vi "Autonomous_Execution.vi"(8 "error in":errorcluster, 9 "Autonomous_Queue":refnum<queue>, 11 "Queue Key":refnum<queue>) -> (2 "Done":bool)   [LabVIEW 2018]
uses:
  Autonomous Utilities/Queue_Key_Data.ctl
  Autonomous Utilities/Robot_Subsystems.ctl
  Subsytems/Drive/Drive_Notifier.ctl
  Subsytems/Drive/Drive_Control_Type.ctl
  Subsytems/Elevator/Elevator_Notifier.ctl
  Subsytems/Elevator/Elevator_Control_Type.ctl
  Subsytems/Elevator/Elevator_Enum_States.ctl
  Subsytems/Climb/Climb_Notifier.ctl
  Subsytems/Climb/Climb_Control_Type.ctl
  Subsytems/Intake_Ball/Intake_Ball_Notifier.ctl
  Subsytems/Intake_Ball/Intake_Ball_Control_Type.ctl
  Subsytems/Intake_Disc/Intake_Disc_Notifier.ctl
  Subsytems/Intake_Disc/Intake_Disc_Control_Type.ctl
  <vilib>/Rock Robotics/WPI/Solenoid/WPI_SolenoidValue.ctl
  Subsytems/Intake_Joint/Intake_Joint_Notifier.ctl
  Subsytems/Intake_Joint/Intake_Joint_Control_Type.ctl
  Subsytems/Intake_Joint/Intake_Joint_Enum_States.ctl
  Global_Variables/Drive_Globals.vi
  Global_Variables/Climb_Globals.vi
  Global_Variables/Elevator_Globals.vi
  Global_Variables/Intake_Joint_Globals.vi
  Global_Variables/Intake_Ball_Globals.vi
  Global_Variables/Intake_Disc_Globals.vi
panel:
  in  "ignore previous (F)":bool
  in  "timeout in ms (-1)":i32=15
  out "notifiers out":refnum<notifier>[](array[refnum])
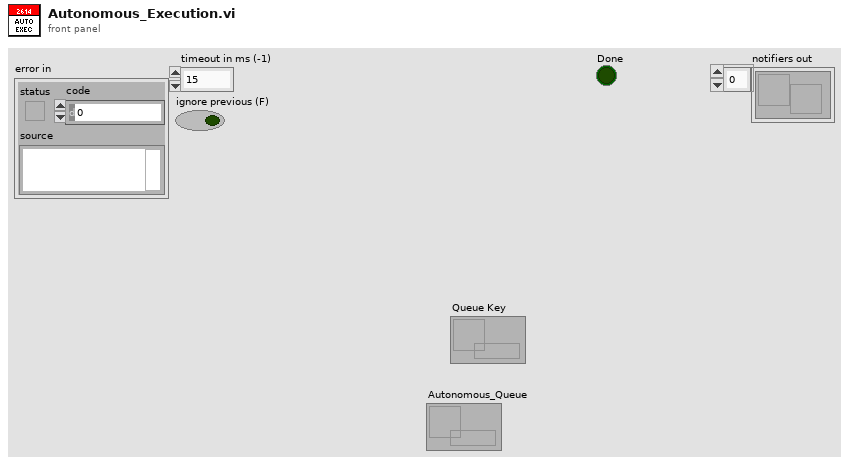
[diagram p1: front panel]
types:
  T1 = typedef "Queue_Key_Data.ctl" = cluster{"Operation Notifier":refnum<notifier>, "Subsystem":string, "Concurrent":bool}
  T2 = typedef "Robot_Subsystems.ctl" = cluster{"Drive Notifier":T3, "Elevator_Notifier":T5, "Climb_Notifier":T8, "Intake_Ball_Notifier":T10, "Intake_Disc_Notifier":T12, "Intake_Joint_Notifier":T15}
  T3 = typedef "Drive_Notifier.ctl" = cluster{"Drive Control List":T4, "Front/Back":dbl, "Left/Right":dbl, "Turn":dbl, "Test_Joy_Y":dbl, "Test_Joy_X":dbl, "Set Wheel Encoder Positions":bool, "Robotcentric":bool, "Reset Gyro":bool, "Rotate Front Right":bool, "Rotate Front Left":bool, "Rotate Back Right":bool, "Rotate Back Left":bool, "Write_Encoder_Positions":bool, "Climb_Advance":bool, "Parameter_One":dbl, "Parameter_Two":dbl, "Parameter_Three":dbl, "Parameter_Four":dbl, "Drive_Notifier":refnum<notifier>, "Step":i32, "Climb_Reverse":bool, "Auto_Target":bool}
  T4 = typedef "Drive_Control_Type.ctl" = enum16{"No_Op", "Write_FL_Position", "Write_FR_Position", "Write_BL_Position", "Write_BR_Position", "Set_Encoder_Positions", "Fieldcentric_PercentVBus", "Fieldcentric", "Robotcentric", "Reset_Gyro", "FR_Wheel", "FL_Wheel", "BR_Wheel", "BL_Wheel", "Drive_Onto_Platform", "Manual_Wheel_Control", "Distance", "Turn_To_Heading", "Turn_To_Target", "Drive_To_Target", "Zero", "Auto_Target", "Drive_Over_Platform", "Heading_Lock", "Time"}
  T5 = typedef "Elevator_Notifier.ctl" = cluster{"Elevator_Control_Type":T6, "Shift":bool, "Brake":bool, "Manual_Lift_Up":bool, "Manual_Lift_Down":bool, "Climb_Advance":bool, "Climb_Reverse":bool, "Low_Rocket":bool, "Mid_Rocket":bool, "High_Rocket":bool, "Cargo_Ship":bool, "Hatch_Floor":bool, "Cargo_Floor":bool, "HP_Hatch":bool, "HP_Cargo":bool, "Depot_Cargo":bool, "Stow":bool, "Set_Position":T7, "Intake_Mode":bool, "Climb_Distance":dbl, "Level_Two":bool, "Parameter_One":dbl, "Parameter_Two":dbl, "Parameter_Three":dbl, "Step":i32, "Elevator_Notifier":refnum<notifier>, "Brake_State":bool, "Shift_State":bool}
  T6 = typedef "Elevator_Control_Type.ctl" = enum16{"No_Op", "Shift", "Brake", "Manual_Elevator_Up", "Manual_Elevator_Down", "Manual_Climb_Up", "Manual_Climb_Down", "Manual_Position_Control", "Elevator_Retract", "Elevator_Extend", "Brake_In_Climb", "Position_Control", "Position", "Shift_Climb"}
  T7 = typedef "Elevator_Enum_States.ctl" = enum16{"Current_Position", "High_Rocket_Hatch_Panel_Floor", "High_Rocket_Hatch_Panel", "Mid_Rocket_Hatch_Panel_Floor", "Mid_Rocket_Hatch_Panel", "Low_Rocket_Hatch_Panel", "Cargo_Ship_Hatch_Panel", "Loading_Station_Hatch_Panel", "Ground_Pickup_Hatch_Panel", "High_Rocket_Cargo", "Mid_Rocket_Cargo", "Low_Rocket_Cargo", "Cargo_Ship_Cargo", "Loading_Station_Cargo", "Ground_Pickup_Cargo", "Depot_Pickup_Cargo", "Descend_Off_Platform", "Stow_Cargo"}
  T8 = typedef "Climb_Notifier.ctl" = cluster{"Climb_Control_Type":T9, "Brake":bool, "Manual_Climb_Up":bool, "Manual_Drive_Forward":bool, "Manual_Drive_Backward":bool, "Manual_Climb_Down":bool, "Climb_Advance":bool, "Climb_Reverse":bool, "Parameter_One":dbl, "Parameter_Two":dbl, "Parameter_Three":dbl, "Step":i32, "Climb_Notifier":refnum<notifier>, "Climb_Distance":dbl, "Level_Two":bool, "Brake_State":bool, "Toggle_Servo":bool}
  T9 = typedef "Climb_Control_Type.ctl" = enum16{"No_Op", "Brake", "Manual_Climb_Up", "Manual_Climb_Down", "Manual_Drive_Forward", "Manual_Drive_Backward", "Back_Wheels_Forward", "Lift_Retract", "Lift_Extend", "Extend_to_Second_Level", "Spin"}
  T10 = typedef "Intake_Ball_Notifier.ctl" = cluster{"Intake_Ball_Control_Type":T11, "Manual_In":bool, "Manual_Out":bool, "Ball_In":bool, "Ball_Out":bool, "Parameter_One":dbl, "Parameter_Two":dbl, "Parameter_Three":dbl, "Step":i32, "Ball_Notifier":refnum<notifier>}
  T11 = typedef "Intake_Ball_Control_Type.ctl" = enum16{"No_Op", "Manual_In", "Manual_Out", "In_Sensor_Stop", "Out_Teleop", "Out", "Stall"}
  T12 = typedef "Intake_Disc_Notifier.ctl" = cluster{"Intake_Disc_Control_Type":T13, "Manual_Disc_Toggle":bool, "Disc_Toggle":bool, "Disc_Toggle_State":bool, "Manual_Press_Toggle":bool, "Disc_Press_State":bool, "Press_Toggle":bool, "Press_Pnuematic":T14, "Disc_Pnuematic":T14, "Disc_Notifier":refnum<notifier>, "Step":i32}
  T13 = typedef "Intake_Disc_Control_Type.ctl" = enum16{"No_Op", "Manual_Disc_Toggle", "Disc_Toggle", "Manual_Press_Toggle", "Press_Toggle", "Acquire_Hatch", "Retract"}
  T14 = typedef "WPI_SolenoidValue.ctl" = enum16{"Off", "On", "Forward", "Reverse"}
  T15 = typedef "Intake_Joint_Notifier.ctl" = cluster{"Intake_Joint_Control_Type":T16, "Manual_Joint_Up":bool, "Manual_Joint_Down":bool, "Low_Rocket":bool, "Mid_Rocket":bool, "High_Rocket":bool, "Cargo_Ship":bool, "Hatch_Floor":bool, "Cargo_Floor":bool, "HP_Hatch":bool, "HP_Cargo":bool, "Depot_Cargo":bool, "Stow":bool, "Intake_Mode":bool, "Set Position":T17, "Parameter_One":dbl, "Parameter_Two":dbl, "Parameter_Three":dbl, "Step":i32, "Joint_Notifier":refnum<notifier>}
  T16 = typedef "Intake_Joint_Control_Type.ctl" = enum16{"No_Op", "Manual_Joint_Up", "Manual_Joint_Down", "Manual_Position_Control", "Position_Control", "Position"}
  T17 = typedef "Intake_Joint_Enum_States.ctl" = enum16{"Current_Position", "High_Rocket_Hatch_Panel_Floor", "High_Rocket_Hatch_Panel", "Mid_Rocket_Hatch_Panel_Floor", "Mid_Rocket_Hatch_Panel", "Low_Rocket_Hatch_Panel", "Cargo_Ship_Hatch_Panel", "Loading_Station_Hatch_Panel", "Ground_Pickup_Hatch_Panel", "High_Rocket_Cargo", "Mid_Rocket_Cargo", "Low_Rocket_Cargo", "Cargo_Ship_Cargo", "Loading_Station_Cargo", "Ground_Pickup_Cargo", "Depot_Pickup_Cargo", "Stow_Cargo", "Get_Hatch"}
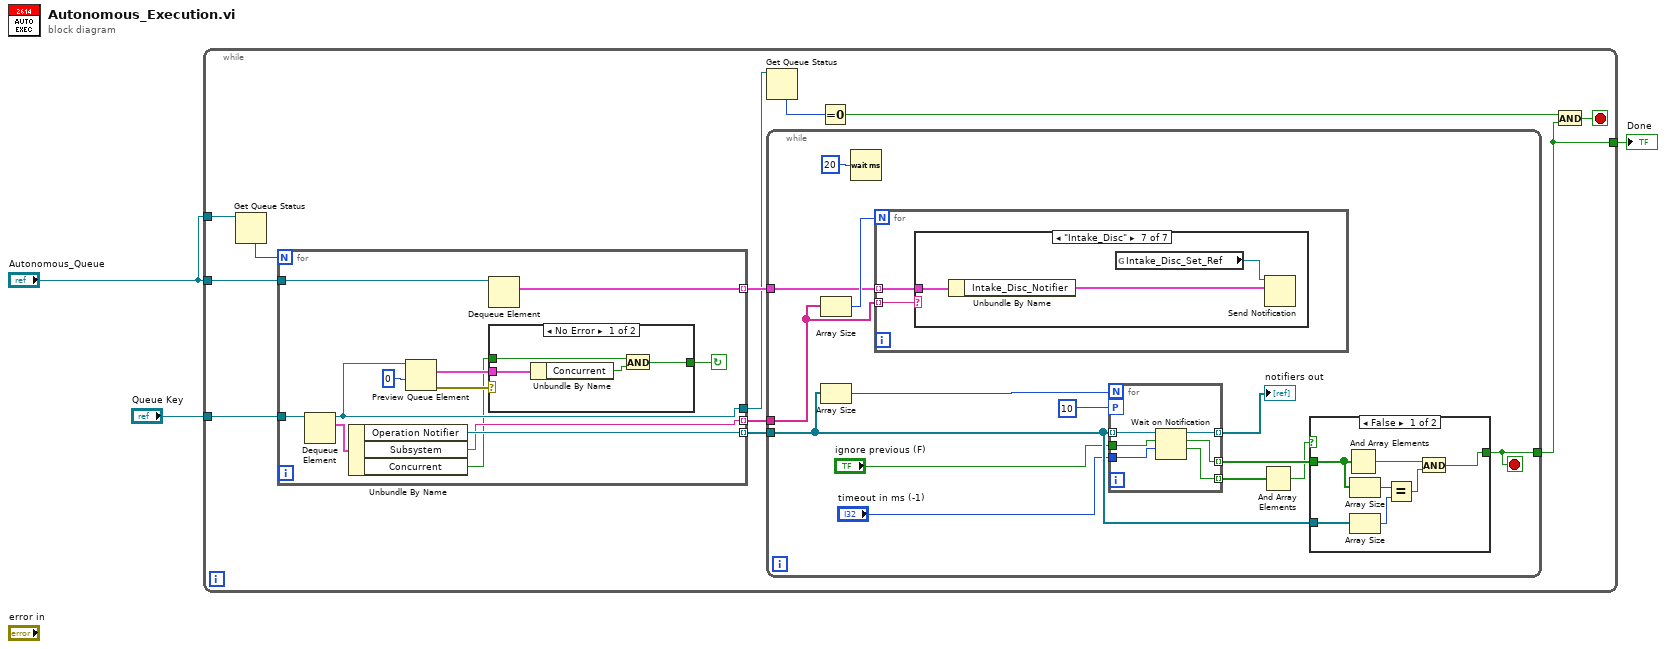
[diagram p0: block diagram]
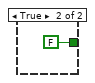
[diagram p2: hidden frame]
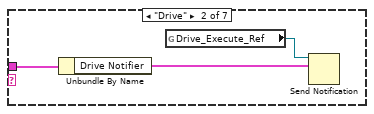
[diagram p4: hidden frame]
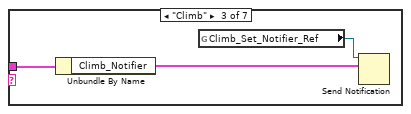
[diagram p5: hidden frame]
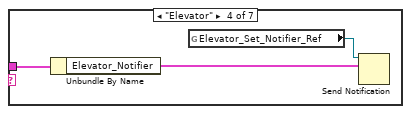
[diagram p6: hidden frame]
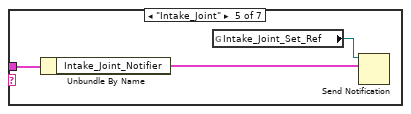
[diagram p7: hidden frame]
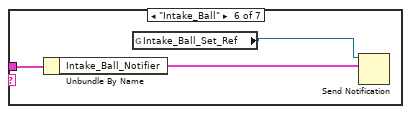
[diagram p8: hidden frame]
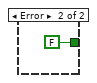
[diagram p9: hidden frame]
diagram:
  n1 = while {
    tunnel: "Queue Key" -> [w14]
    tunnel: "Autonomous_Queue" -> [w15]
    tunnel: "Autonomous_Queue" -> [w6]
    tunnel: [w4] -> w1
    stop <- w7 stop-if-true
    n2 = Get Queue Status(queue=w6) -> (# elements in queue=w9:i32)  [unwired: 2 in, 7 out]
    n3 = for {
      N: w9 -> [_]
      tunnel: w15 -> [w69]
      tunnel: w14 -> [w75]
      tunnel: [w66] -> w10 mode=indexing
      tunnel: [w70] -> w5
      tunnel: [w65] -> w12 mode=indexing
      tunnel: [w68] -> w11 mode=indexing
      stop <- w71 continue-if-true
      n4 = Dequeue Element(queue=w75) -> (queue out=w70:refnum<queue>, element=w67:T1)  [unwired: 2 in, 2 out]
      n5 = Unbundle By Name(w67) -> ("Operation Notifier"=w66:refnum<notifier>, "Subsystem"=w65:string, "Concurrent"=w64:bool)
      n6 = Preview Queue Element(queue=w70, timeout in ms (-1)=0) -> (element=w74:T1, error out=w72:errorcluster)  [unwired: 1 in, 2 out]
      n7 = Dequeue Element(queue=w69) -> (element=w68:T2)  [unwired: 2 in, 3 out]
      n8 = case shown="No Error" w72 {
        tunnel: w74 -> [w77 _]
        tunnel: [w79 FALSE] -> w71
        tunnel: w64 -> [w78 _]
        frame No Error {
          n9 = Unbundle By Name(w77) -> ("Concurrent"=w76:bool)
          n10 = And(x=w78, y=w76) -> (x .and. y?=w79:bool)
        }
        frame Error {
        }
      }
    }
    n11 = Get Queue Status(queue=w5) -> (# elements in queue=w13:i32)  [unwired: 2 in, 7 out]
    n12 = while {
      tunnel: w12 -> [w24]
      tunnel: w11 -> [w23]
      tunnel: w10 -> [w25]
      tunnel: [w26] -> w4
      stop <- w26 stop-if-true
      n13 = Array Size(array=w24) -> (size(s)=w27:i32)
      n14 = Array Size(array=w25) -> (size(s)=w19:i32)
      n15 = Wait (ms)(milliseconds to wait=u32 20) -> ()  [unwired: 1 out]
      n16 = for {
        N: w27 -> [_]
        tunnel: w24 -> [w45] mode=indexing
        tunnel: w23 -> [w44] mode=indexing
        n17 = case shown="\"Intake_Disc\"" w45 {
          tunnel: w44 -> [_ w47 w50 w54 w57 w60 w63]
          frame "No_Op", Default {
          }
          frame "Drive" {
            n18 = Unbundle By Name(w47) -> ("Drive Notifier"=w46:T3)
            n19 = global read "Drive_Globals.vi" "Drive_Execute_Ref"() -> (w48:refnum<notifier>)
            n20 = Send Notification(notification=w46, notifier=w48) -> ()  [unwired: 1 in, 2 out]
          }
          frame "Climb" {
            n21 = Unbundle By Name(w50) -> ("Climb_Notifier"=w51:T8)
            n22 = global read "Climb_Globals.vi" "Climb_Set_Notifier_Ref"() -> (w49:refnum<notifier>)
            n23 = Send Notification(notification=w51, notifier=w49) -> ()  [unwired: 1 in, 2 out]
          }
          frame "Elevator" {
            n24 = Unbundle By Name(w54) -> ("Elevator_Notifier"=w53:T5)
            n25 = global read "Elevator_Globals.vi" "Elevator_Set_Notifier_Ref"() -> (w52:refnum<notifier>)
            n26 = Send Notification(notification=w53, notifier=w52) -> ()  [unwired: 1 in, 2 out]
          }
          frame "Intake_Joint" {
            n27 = Unbundle By Name(w57) -> ("Intake_Joint_Notifier"=w56:T15)
            n28 = global read "Intake_Joint_Globals.vi" "Intake_Joint_Set_Ref"() -> (w55:refnum<notifier>)
            n29 = Send Notification(notification=w56, notifier=w55) -> ()  [unwired: 1 in, 2 out]
          }
          frame "Intake_Ball" {
            n30 = Unbundle By Name(w60) -> ("Intake_Ball_Notifier"=w59:T10)
            n31 = global read "Intake_Ball_Globals.vi" "Intake_Ball_Set_Ref"() -> (w58:refnum<notifier>)
            n32 = Send Notification(notification=w59, notifier=w58) -> ()  [unwired: 1 in, 2 out]
          }
          frame "Intake_Disc" {
            n33 = Unbundle By Name(w63) -> ("Intake_Disc_Notifier"=w62:T12)
            n34 = global read "Intake_Disc_Globals.vi" "Intake_Disc_Set_Ref"() -> (w61:refnum<notifier>)
            n35 = Send Notification(notification=w62, notifier=w61) -> ()  [unwired: 1 in, 2 out]
          }
        }
      }
      n36 = for {
        N: w19 -> [_]
        tunnel: w25 -> [w35] mode=indexing
        workers-P: 10 -> [_]
        tunnel: "timeout in ms (-1)" -> [w34]
        tunnel: "ignore previous (F)" -> [w33]
        tunnel: [w32] -> w22 mode=indexing
        tunnel: [w31] -> w29 mode=indexing
        tunnel: [w30] -> w17 mode=indexing
        n37 = Wait on Notification(notifier=w35, ignore previous (F)=w33, timeout in ms (-1)=w34) -> (notifier out=w32:refnum<notifier>, notification=w31:bool, timed out?=w30:bool)  [unwired: 1 in, 1 out]
      }
      "notifiers out" <- w22
      n38 = And Array Elements(Boolean array=w17) -> (logical AND=w28:bool)
      n39 = case shown="False" w28 {
        tunnel: [w41 FALSE] -> w26
        tunnel: w29 -> [w40 _]
        tunnel: w25 -> [w39 _]
        frame False {
          n40 = And Array Elements(Boolean array=w40) -> (logical AND=w42:bool)
          n41 = Array Size(array=w40) -> (size(s)=w38:i32)
          n42 = Array Size(array=w39) -> (size(s)=w37:i32)
          n43 = Equal?(x=w38, y=w37) -> (x = y?=w36:bool)
          n44 = And(x=w42, y=w36) -> (x .and. y?=w41:bool)
        }
        frame True {
        }
      }
    }
    n45 = Equal To 0?(x=w13) -> (x = 0?=w8:bool)
    n46 = And(x=w8, y=w4) -> (x .and. y?=w7:bool)
  }
  "Done" <- w1
